vi "string_to_paragraph.vi"(8 "error in (no error)":errorcluster, 10 "no_of_char":i32=70, 11 "string in":string) -> (0 "error out":errorcluster, 3 "string out":string)   [LabVIEW 2015, in "lv-dialog-interfaces.lvlib"]
doc: "this will take a given string and truncate it such that each line has a maximum of the given number of characters breaking lines on whitespace."
uses:
  lv-dialog-interfaces.lvlib
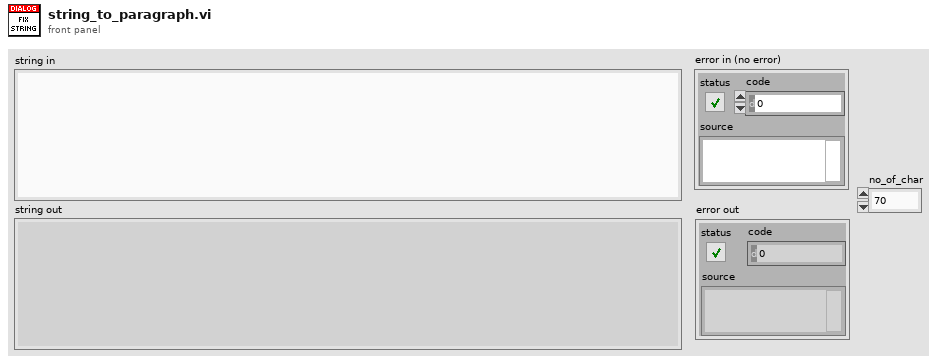
[diagram p1: front panel]
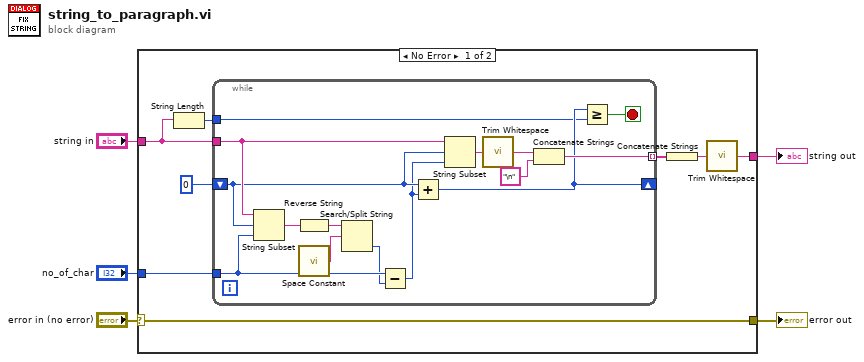
[diagram p0: block diagram]
diagram:
  n1 = case shown="No Error" "error in (no error)" {
    selector: "error in (no error)" -> [w6 w29]
    tunnel: "string in" -> [w13 _]
    tunnel: [w12 _] -> w4
    tunnel: "no_of_char" -> [w8 _]
    tunnel: [w6 w29] -> w1
    frame No Error {
      n2 = String Length(string=w13) -> (length=w7:i32)
      n3 = while {
        tunnel: w8 -> [w25]
        shift-right: [w16] -> _
        shift-left: 0 -> [w22]
        tunnel: w13 -> [w23]
        tunnel: [w17] -> w10 mode=indexing
        tunnel: w7 -> [w14]
        stop <- w15 stop-if-true
        n4 = String Subset(string=w23, offset (0)=w22, length (rest)=w25) -> (substring=w28:string)
        n5 = Reverse String(1:w28) -> (0:w27:string)
        n6 = call <vilib>:"Space Constant.vi"() -> ("String"=w26:string)
        n7 = Search/Split String(string=w27, search string/char (-)=w26) -> (offset of match=w24:i32)  [unwired: 1 in, 2 out]
        n8 = Subtract(x=w25, y=w24) -> (x-y=w21:i32)
        n9 = Add(x=w22, y=w21) -> (x+y=w16:i32)
        n10 = String Subset(string=w23, offset (0)=w22, length (rest)=w21) -> (substring=w20:string)
        n11 = call <vilib>:"Trim Whitespace.vi"("string"=w20) -> ("trimmed string"=w19:string)  [unwired: 1 in]
        n12 = Concatenate Strings(w19, "\n") -> (w17:string)
        n13 = Greater Or Equal?(x=w16, y=w14) -> (x >= y?=w15:bool)
      }
      n14 = Concatenate Strings(w10) -> (w9:string)
      n15 = call <vilib>:"Trim Whitespace.vi"("string"=w9) -> ("trimmed string"=w12:string)  [unwired: 1 in]
    }
    frame Error {
    }
  }
  "string out" <- w4
  "error out" <- w1
